vi "TC560-Release.vi"(8 "error in":errorcluster, 11 "VISA Resource Name":refnum<visa-resource-name>) -> (0 "error out":errorcluster)   [LabVIEW 2018]
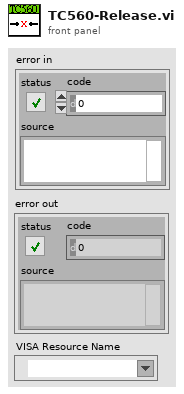
[diagram p1: front panel]
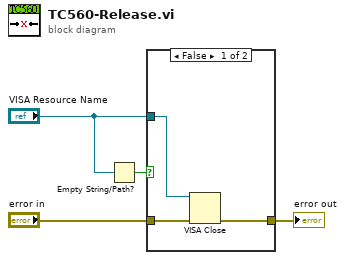
[diagram p0: block diagram]
diagram:
  n1 = Empty String/Path?(string/path="VISA Resource Name") -> (empty?=w4:bool)
  n2 = case shown="False" w4 {
    tunnel: "VISA Resource Name" -> [w6 _]
    tunnel: "error in" -> [w7 w8]
    tunnel: [w5 w8] -> w1
    frame False {
      n3 = VISA Close(VISA resource name=w6, error in (no error)=w7) -> (error out=w5:errorcluster)
    }
    frame True {
    }
  }
  "error out" <- w1
